vi "_File Exists__ogtk.vi"   [LabVIEW 2020, in "Global_logger.lvlib"]
doc: "Checks to see whether a path exists on disk and whether it is a directory."
uses:
  Global_logger.lvlib
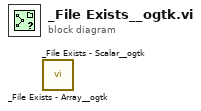
[diagram p0: block diagram]
diagram:
  n1 = call "_File Exists - Array__ogtk.vi"() -> ()  [unwired: 7 in, 2 out]
  n2 = call "_File Exists - Scalar__ogtk.vi"() -> ()  [unwired: 7 in, 2 out]
